vi "Read Launch Position.vi"(11 "Philips Dialog in":refnum<class "Flex UI Dialog.lvclass">) -> (2 "Launch Position":T1, 3 "Philips Dialog out":refnum<class "Flex UI Dialog.lvclass">)   [LabVIEW 2014, in "Flex UI Dialog.lvclass"]
uses:
  Flex UI Dialog.lvclass
  Enum - Launch Position.ctl
  Flex UI Dialog.lvclass/Flex UI Dialog.ctl
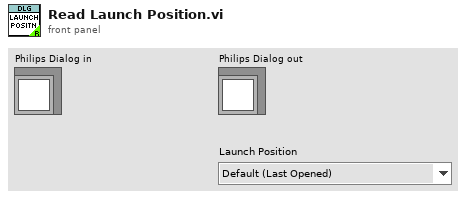
[diagram p1: front panel]
types:
  T1 = typedef "Flex UI Dialog.lvclass/Enum - Launch Position.ctl" = enum16{"Default (Last Opened)", "Centered", "Centered on Caller", "Maximized", "Hidden"}
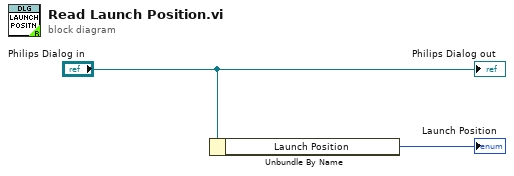
[diagram p0: block diagram]
diagram:
  n1 = Unbundle By Name("Philips Dialog in") -> ("Launch Position"=→"Launch Position":T1)
  "Philips Dialog out" <- "Philips Dialog in"
